vi "Stop Core.vi"(10 "final error code":i32, 11 "BNT_ULx-MCSV-DOPWM in":refnum<class "BNT_ULx-MCSV-DOPWM.lvclass">) -> (3 "BNT_ULx-MCSV-DOPWM out":refnum<class "BNT_ULx-MCSV-DOPWM.lvclass">)   [LabVIEW 2021, in "BNT_ULx.lvlib" / "BNT_ULx-MCSV-DOPWM.lvclass"]
doc: "(<B>Filename</B>: Actor Framework.lvlib:Actor.lvclass:Stop Core.vi)\n\nDefines what the actor does before it stops. Use the <B>final error code</B> input to determine whether the actor shut down in response to an error.\n\nBy default, this method does nothing. A descendant class may override it to define behavior, such as shutting down any processes the actor initiated in its override of the Actor Core method."
uses:
  BNT_ULx-MCSV-DOPWM.lvclass
  BNT_ULx-MCSV-DOPWM.lvclass/BNT_ULx-MCSV-DOPWM.ctl
  BNT_ULx-MCSV/BNT_ULx-MCSV.lvclass
  CSPP_Core/Classes/CSPP_ProcessVariables/PVConnection/PVConnection.lvclass
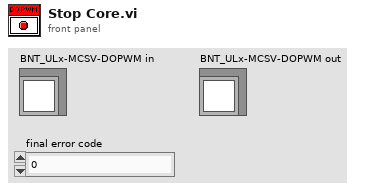
[diagram p1: front panel]
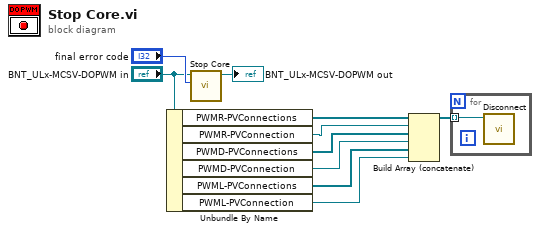
[diagram p0: block diagram]
diagram:
  n1 = Unbundle By Name("BNT_ULx-MCSV-DOPWM in") -> ("PWMR-PVConnections"=w7:refnum<class "PVConnection.lvclass">[], "PWMR-PVConnection"=w5:refnum<class "PVConnection.lvclass">, "PWMD-PVConnections"=w4:refnum<class "PVConnection.lvclass">[], "PWMD-PVConnection"=w3:refnum<class "PVConnection.lvclass">, "PWML-PVConnections"=w2:refnum<class "PVConnection.lvclass">[], "PWML-PVConnection"=w1:refnum<class "PVConnection.lvclass">)
  n2 = call-parent "Stop Core.vi"("final error code"="final error code", "BNT_ULx-MCSV in"="BNT_ULx-MCSV-DOPWM in") -> ("BNT_ULx-MCSV out"=→"BNT_ULx-MCSV-DOPWM out":refnum<class "BNT_ULx-MCSV-DOPWM.lvclass">)  [unwired: 9 in]
  n3 = Build Array (concatenate)(w7, w5, w4, w3, w2, w1) -> (w6:refnum<class "PVConnection.lvclass">[])
  n4 = for {
    tunnel: w6 -> [w11] mode=indexing
    n5 = call "Disconnect.vi"("PVConnection in"=w11) -> ()  [unwired: 9 in, 2 out]
  }
